vi "FindAllChildrenOf.vi"(10 "Name":string, 11 "RelationshipBrowser":refnum<class "IRelationshipBrowser.lvclass">) -> (3 "Children":refnum<class "Person.lvclass">[](array[class]))   [LabVIEW 2018, in "IRelationshipBrowser.lvclass"]
uses:
  IRelationshipBrowser.lvclass
  Person/Person.lvclass
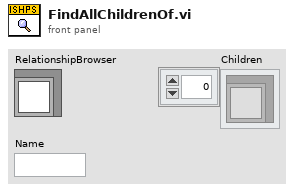
[diagram p1: front panel]
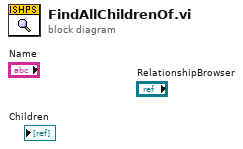
[diagram p0: block diagram]
diagram:
